vi "FPGA Read Back Sensor.vi"(1 "stop":bool) -> (0 "Time of Flight":u32)   [LabVIEW 2015]
uses:
  <vilib>/rvi/Emulation/niFpgaGetClockAttributes.vi
  <vilib>/rvi/Emulation/niFpgaSctlEmulationGetInTimedLoop.vi
  <vilib>/rvi/Emulation/niFpgaEmulationReportErrorSimple.vi
  <vilib>/rvi/eio/common/nirviEmuTemplateMethod_errors.vi
  <vilib>/rvi/Emulation/niFpgaCriticalErrorInLSC.vi
  <vilib>/rvi/Emulation/niFpgaProcessEmulError.vi
  <vilib>/eio/EIONode/EIONode.xnode
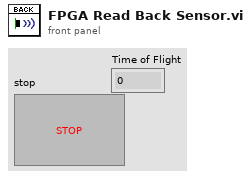
[diagram p1: front panel]
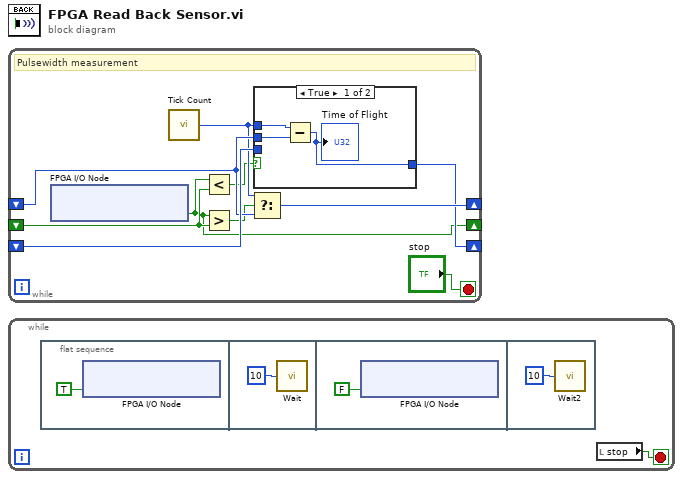
[diagram p0: block diagram]
diagram:
  n1 = while "Pulsewidth Measurement + Sound Output" {
    shift-left: _ -> [w10]
    shift-right: [w5] -> _
    shift-left: _ -> [w9]
    shift-right: [w8] -> _
    shift-left: _ -> [w6]
    shift-right: [w2] -> _
    stop <- "stop" stop-if-true
    # "Pulsewidth measurement"
    n2 = xnode "FPGA I/O Node"() -> ("ConnectorB/DIO1"=w2:bool)  [unwired: 1 in, 1 out]
    n3 = call "Tick Count"() -> ("Tick Count(uSec)"=w4:u32)
    n4 = Less?(x=w2, y=w6) -> (x < y?=w3:bool)
    n5 = Greater?(x=w2, y=w6) -> (0:w7:bool)
    n6 = Select(t=w4, s=w7, f=w9) -> (s? t:f=w8:u32)
    n7 = case shown="True" w3 {
      tunnel: w10 -> [_ w14]
      tunnel: w4 -> [w12 _]
      tunnel: w9 -> [w13 _]
      tunnel: [w11 w14] -> w5
      frame True {
        n8 = Subtract(x=w12, y=w13) -> (x-y=w11:u32)
        "Time of Flight" <- w11
      }
      frame False {
      }
    }
  }
  n9 = while {
    stop <- w15 stop-if-true
    n10 = flat-sequence {
      frame #0 {
        n11 = xnode "FPGA I/O Node"("ConnectorB/DIO2"=TRUE ("ConnectorB/DIO4")) -> ()  [unwired: 1 in, 1 out]
      }
      frame #1 {
        n12 = call "Wait"("Count(uSec)"=u32 10 ("Count(mSec)")) -> ()  [unwired: 1 out]
      }
      frame #2 {
        n13 = xnode "FPGA I/O Node"("ConnectorB/DIO2"=FALSE ("ConnectorB/DIO4")) -> ()  [unwired: 1 in, 1 out]
      }
      frame #3 {
        n14 = call "Wait2"("Count(mSec)"=u32 10) -> ()  [unwired: 1 out]
      }
    }
    n15 = local read "stop"() -> (w15:bool)
  }
